vi "Main.vi"() -> ()   [LabVIEW 2021]
uses:
  system/mode.ctl
  <vilib>/Platform/TimedLoop/XDataNode/timing_clust.ctl
  <vilib>/Platform/TimedLoop/XDataNode/nitl_modes.ctl
  <vilib>/Platform/TimedLoop/XDataNode/wakeup.ctl
  <vilib>/Platform/TimedLoop/XDataNode/XDataNode.xnode
  system/System.lvclass
  <vilib>/Platform/TimedLoop/XDataNode/XDNodeRunTimeDep.lvlib
panel:
  in  "Dynamic scaler : FBLR":dbl[](array[numeric])=[0.0, 0.0, 0.0, 0.0]
  in  "Dynamic scaler : pry":dbl[](array[numeric])=[0.0, 0.0, 0.0]
  out "Elapsed Time":dbl
  out "Sample Idx":dbl
  out "Iteration Duration":dbl
  out "F - B - L - R":dbl[](array[numeric])
  in  "mode":T1=enum."pry_CL"
  in  "Period":u32=50
  out "RST path":path
  in  "RST":path=path "yawSolo"
  out "Refs loc":path
  out "Output loc":path
  in  "Output file":path=path "trash"
  in  "Refs file":path=path "onesA"
  out "MotorInputs":T2(graph)
  out "error":errorcluster
  in  "stop":bool
  out "AngleOutputs":T3(graph)
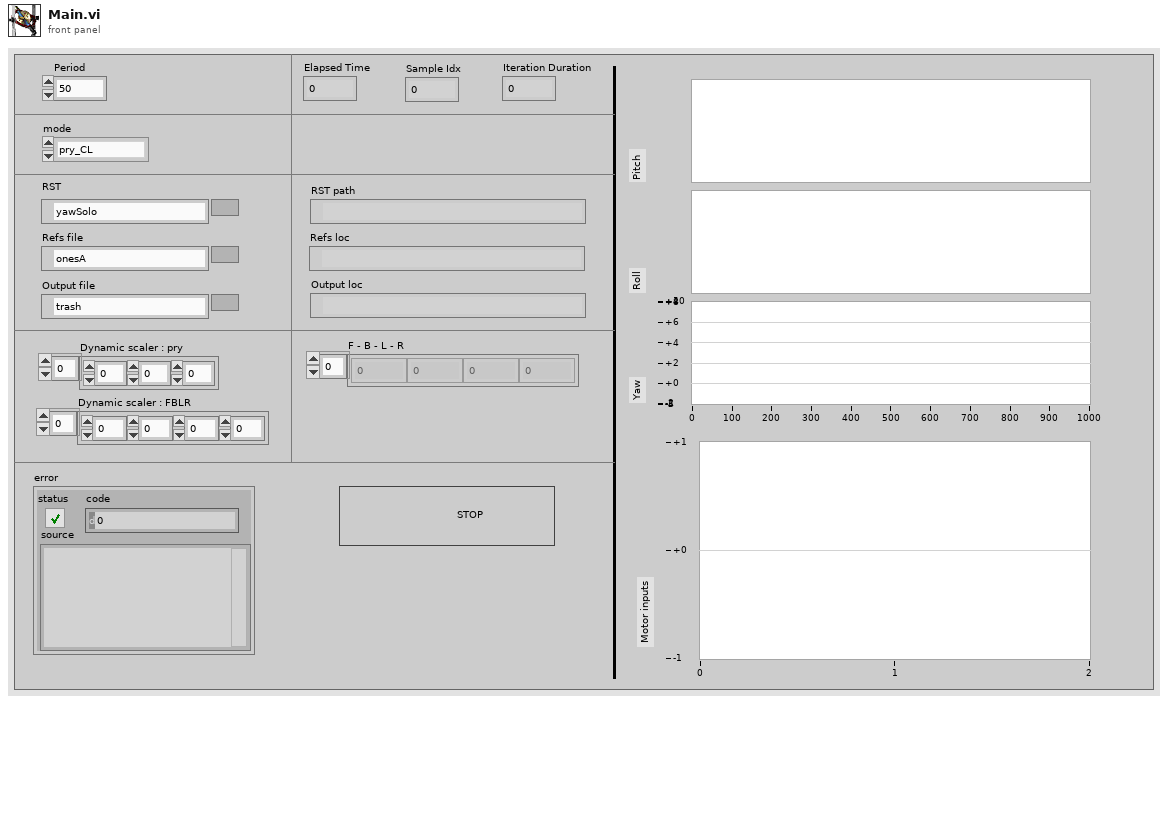
[diagram p1: front panel]
types:
  T1 = typedef "System.lvclass/mode.ctl" = enum16{"pry_OL", "pry_CL", "FBLR_CL"}
  T2 = cluster{"Unstacked Array[0]":dbl, "Unstacked Array[1]":dbl, "Unstacked Array[2]":dbl, "Unstacked Array[3]":dbl}
  T3 = cluster{"Unstacked Array[0]":dbl, "Unstacked Array[1]":dbl, "Unstacked Array[2]":dbl}
  T4 = typedef "XDNodeRunTimeDep.lvlib/timing_clust.ctl" = cluster{"Expected End [f-1]":u64, "Actual End [f-1]":u64, "Finished Late? [f-1]":bool, "Expected End [i-1]":u64, "Actual End [i-1]":u64, "Finished Late? [i-1]":bool, "Expected Start [i]":u64, "Actual Start [i]":u64, "Expected Start [f]":u64, "Actual Start [f]":u64, "Source Name":string, "Structure Name":string, "Period":i64, "Deadline":i64, "Offset":i64, "Start":i64, "Priority":i32, "Timeout":i32, "Mode":T5, "Wakeup Reason":T6, "Error":errorcluster, "Source Type":string, "Secondary Source Type":string, "Global End Time":u64, "Global Start Time":u64, "Frame Duration":u64, "Iteration Duration":u64, "Assigned CPU":i32, "I/O Scan Engine Mode":u32}
  T5 = typedef "XDNodeRunTimeDep.lvlib/nitl_modes.ctl" = enum32{"No Change", "Process missed periods, maintain original phase", "Discard missed periods, maintain original phase", "Process missed periods, ignore original phase", "Discard missed periods, ignore original phase"}
  T6 = typedef "XDNodeRunTimeDep.lvlib/wakeup.ctl" = enum32{"Normal", "Aborted", "Asynchronous wakeup", "Timing source error", "Timed loop error", "Timeout"}
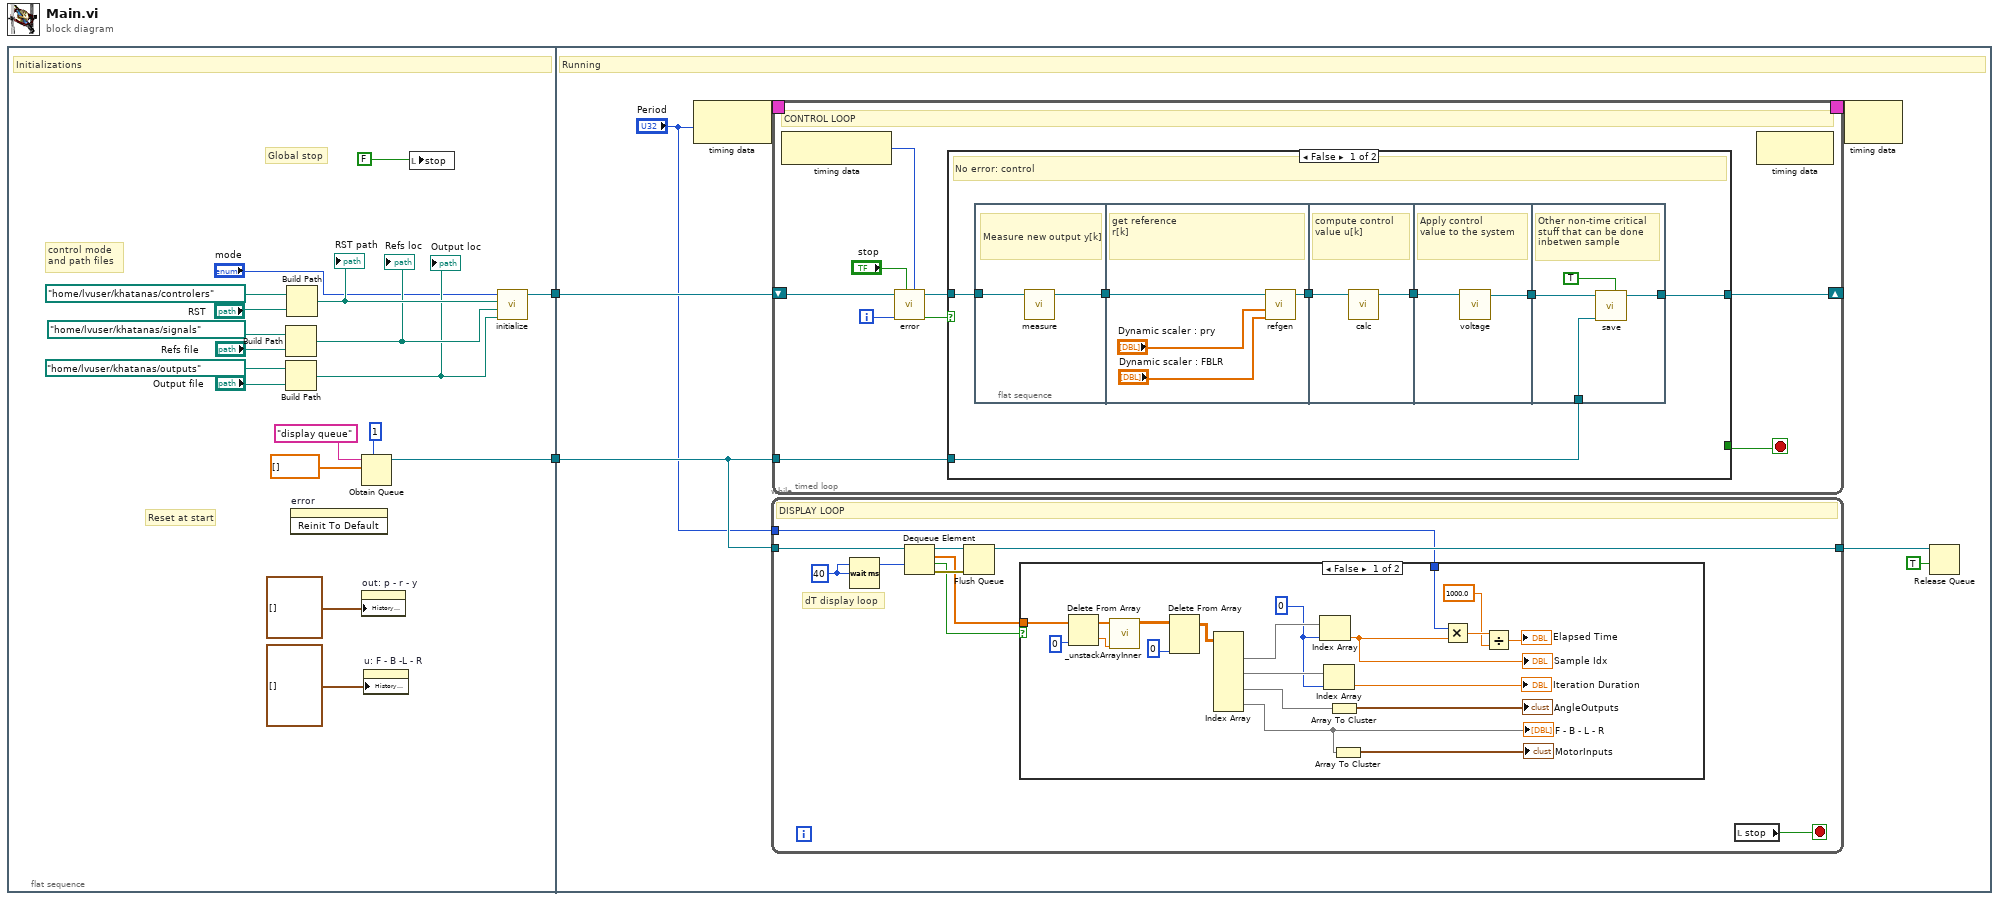
[diagram p0: block diagram]
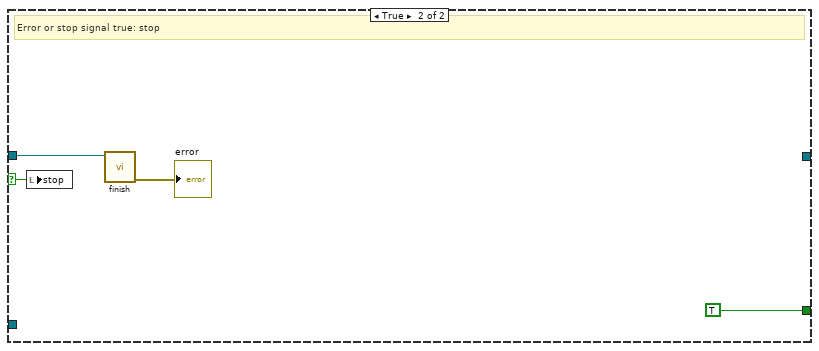
[diagram p2: hidden frame]
diagram:
  n1 = flat-sequence {
    tunnel: [w16] -> w2
    tunnel: [w20] -> w1
    tunnel: w2 -> [w23]
    tunnel: w1 -> [w22]
    frame #0 {
      # "control mode \nand path files"
      # "Reset at start"
      # "Global stop"
      # "Initializations"
      n2 = Build Path(base path=path "/home/lvuser/khatanas/signals", name or relative path="Refs file") -> (appended path=w5:path)
      "Refs loc" <- w5
      n3 = Build Path(base path=path "/home/lvuser/khatanas/outputs", name or relative path="Output file") -> (appended path=w4:path)
      "Output loc" <- w4
      n4 = Build Path(base path=path "/home/lvuser/khatanas/controlers", name or relative path="RST") -> (appended path=w6:path)
      "RST path" <- w6
      n5 = invoke on="error" class="Clust (strict)" method="Reinit To Default"() -> ()  [unwired: 3 in, 3 out]
      n6 = Obtain Queue(max queue size (-1, unlimited)=1, name (unnamed)="display queue", element data type=dbl[] [] ("y")) -> (queue out=w20:refnum<queue>)  [unwired: 2 in, 2 out]
      n7 = property on="out: p - r - y" class="WFChart (strict)"("History Data"=cluster{"y":dbl, "y":dbl, "y":dbl}[] []) -> ()  [unwired: 2 in, 2 out]
      n8 = property on="u: F - B -L - R" class="WFChart (strict)"("History Data"=cluster{"y":dbl, "y":dbl, "y":dbl, "y 2":dbl}[] []) -> ()  [unwired: 2 in, 2 out]
      n9 = local write "stop"(FALSE ("stop")) -> ()
      n10 = call "initialize.vi"("Data Savefile Path"=w4, "Refs Readfrom Path"=w5, "RST Readfrom path"=w6, "mode"="mode") -> ("Qube"=w16:refnum<class "System.lvclass">)  [unwired: 7 in]
    }
    frame #1 {
      # "Running"
      n11 = node-c288("Period") -> (w27:T4)
      n12 = while {
        tunnel: w22 -> [w76]
        tunnel: [w70] -> w25
        tunnel: "Period" -> [w69]
        stop <- w77 stop-if-true
        w73 = u32 40 ("Ts")
        # "dT display loop"
        # "DISPLAY LOOP"
        n13 = Wait (ms)(milliseconds to wait=w73) -> ()  [unwired: 1 out]
        n14 = Dequeue Element(queue=w76, timeout in ms (-1)=w73) -> (queue out=w75:refnum<queue>, element=w72:dbl[], timed out?=w71:bool, error out=w74:errorcluster)  [unwired: 1 in]
        n15 = Flush Queue(queue=w75, error in (no error)=w74) -> (queue out=w70:refnum<queue>)  [unwired: 2 out]
        n16 = case shown="False" w71 {
          tunnel: w72 -> [w97 _]
          tunnel: w69 -> [w82 _]
          frame False {
            w78 = 0 ("index")
            n17 = Delete From Array(array=w97, index=0) -> (deleted portion=w94:dbl, array with subset deleted=w95:dbl[])  [unwired: 1 in]
            n18 = call "_unstackArrayInner.vi"("#iter"=w94, "Stacked Array"=w95) -> ("Unstacked Array"=w90:dbl[][])  [unwired: 9 in]
            n19 = Delete From Array(array=w90, index (col)=0 ("disabled index (col)")) -> (array with subset deleted=w89:dbl[][])  [unwired: 2 in, 1 out]
            n20 = Index Array(array=w89) -> (element #1=w83:dbl[], element #2=w85:dbl[], element #3=w87:dbl[], element #4=w88:dbl[])  [unwired: 8 in]
            "F - B - L - R" <- w88
            n21 = Index Array(array=w83, index=w78) -> (element=w81:dbl)
            "Sample Idx" <- w81
            n22 = Index Array(array=w85, index=w78) -> (element=→"Iteration Duration":dbl)
            n23 = Array To Cluster(array=w87) -> (cluster=→"AngleOutputs":T3)
            n24 = Array To Cluster(array=w88) -> (cluster=→"MotorInputs":T2)
            n25 = Multiply(x=w82, y=w81) -> (x*y=w80:dbl)
            n26 = Divide(x=w80, y=1000.0) -> (x/y=→"Elapsed Time":dbl)
          }
          frame True {
          }
        }
        n27 = local read "stop"() -> (w77:bool)
      }
      n28 = timed-loop {
        tunnel: w22 -> [w35]
        timing: w27 -> [_]
        timing-out: [_] -> w26
        shift-right: [w31] -> _
        shift-left: w23 -> [w33]
        i -> [w29]
        stop <- w36 stop-if-true
        # "CONTROL LOOP"
        n29 = node-c288() -> (w28:i64)  [unwired: 1 in]
        n30 = call "error.vi"("Iteration duration"=w28, "stop"="stop", "idx"=w29, "Qube"=w33) -> ("abort?"=w34:bool, "Qube"=w30:refnum<class "System.lvclass">)  [unwired: 6 in]
        n31 = case shown="False" w34 {
          selector: w34 -> [_ w62]
          tunnel: w30 -> [w44 w63]
          tunnel: [_ TRUE] -> w36
          tunnel: w35 -> [w40 _]
          tunnel: [w43 _] -> w31
          frame False {
            # "No error: control"
            n32 = flat-sequence {
              tunnel: [w47] -> w42
              tunnel: w44 -> [w48]
              tunnel: w42 -> [w52]
              tunnel: [w51] -> w41
              tunnel: [w54] -> w45
              tunnel: w41 -> [w53]
              tunnel: [w56] -> w46
              tunnel: w45 -> [w55]
              tunnel: w46 -> [w60]
              tunnel: w40 -> [w57]
              tunnel: [w58] -> w43
              frame #0 {
                # "Measure new output y[k]"
                n33 = call "measure.vi"("Qube"=w48) -> ("Qube"=w47:refnum<class "System.lvclass">)  [unwired: 10 in]
              }
              frame #1 {
                # "get reference \nr[k]"
                n34 = call "refgen.vi"("Dynamic scaller: FBLR"="Dynamic scaler : FBLR", "Dynamic scaller: pry"="Dynamic scaler : pry", "Qube"=w52) -> ("Qube"=w51:refnum<class "System.lvclass">)  [unwired: 6 in]
              }
              frame #2 {
                # "compute control value u[k]"
                n35 = call "calc.vi"("Qube"=w53) -> ("Qube"=w54:refnum<class "System.lvclass">)  [unwired: 10 in]
              }
              frame #3 {
                # "Apply control \nvalue to the system"
                n36 = call "voltage.vi"("Qube"=w55) -> ("Qube"=w56:refnum<class "System.lvclass">)  [unwired: 10 in]
              }
              frame #4 {
                # "Other non-time critical stuff that can be done inbetwen sample"
                n37 = call "save.vi"("log?"=TRUE, "queue in"=w57, "Qube"=w60) -> ("Qube"=w58:refnum<class "System.lvclass">)  [unwired: 8 in]
              }
            }
          }
          frame True {
            # "Error or stop signal true: stop"
            n38 = local write "stop"(w62) -> ()
            n39 = call "finish.vi"("ActiveSuspension.lvclass"=w63) -> ("error out"=→"error":errorcluster)  [unwired: 10 in]
          }
        }
        n40 = node-c288() -> ()  [unwired: 1 in, 1 out]
      }
      n41 = node-c288(w26) -> ()  [unwired: 1 out]
      n42 = Release Queue(queue=w25, force destroy? (F)=TRUE) -> ()  [unwired: 1 in, 3 out]
    }
  }
